vi "Data Conversion - Signed 16 Bit Array to Byte Array.vi"(9 "16 Bit Array (Signed) In":i16[](array[numeric]), 10 "Byte Order":T1(ring)) -> (1 "Byte Array (Unsigned) Out":u8[](array[numeric]))   [LabVIEW 2017, in "Communications Library.lvlib"]
doc: "Converts a 16 bit array of integers into a byte array"
uses:
  Communications Library.lvlib
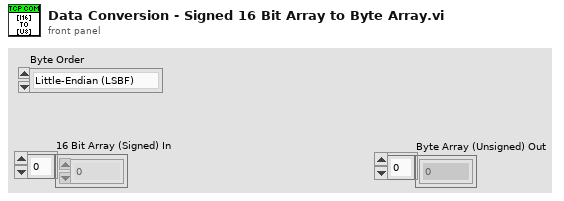
[diagram p1: front panel]
types:
  T1 = enum16{"Little-Endian (LSBF)", "Big-Endian (MSBF)"}
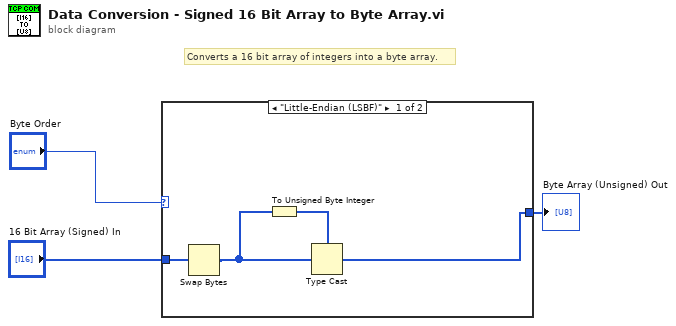
[diagram p0: block diagram]
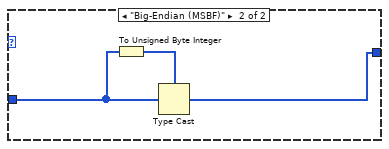
[diagram p2: hidden frame]
diagram:
  # "Converts a 16 bit array of integers into a byte array."
  n1 = case shown="\"Little-Endian (LSBF)\"" "Byte Order" {
    tunnel: "16 Bit Array (Signed) In" -> [w5 w8]
    tunnel: [w6 w9] -> w1
    frame "Little-Endian (LSBF)" {
      n2 = Swap Bytes(anything=w5) -> (byte swapped=w4:i16[])
      n3 = To Unsigned Byte Integer(number=w4) -> (unsigned 8bit integer=w7:u8[])
      n4 = Type Cast(type=w7, x=w4) -> (*(type *) &x=w6:u8[])
    }
    frame "Big-Endian (MSBF)" {
      n5 = To Unsigned Byte Integer(number=w8) -> (unsigned 8bit integer=w10:u8[])
      n6 = Type Cast(type=w10, x=w8) -> (*(type *) &x=w9:u8[])
    }
  }
  "Byte Array (Unsigned) Out" <- w1
